vi "PISetAxisPos.vi"(0 "Position":sgl format="%.2f", 1 "Axis":i32) -> ()   [LabVIEW 2009]
uses:
  AO Update Channel (scaled value).vi
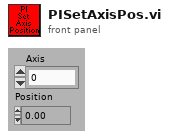
[diagram p1: front panel]
types:
  T1 = typedef "StageSettings.ctt" = cluster{"channels (x, y, z)":tag, "Stage Scaling (V/µm)":dbl}
  T2 = typedef "AnalogSettings.ctt" = cluster{"PCI 671x Device Number":u32, "Samples per Unit":u32}
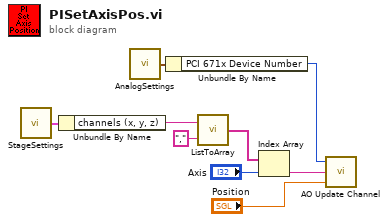
[diagram p0: block diagram]
diagram:
  n1 = call "StageSettings.vi"() -> ("PI Stage Setup (output)"=w9:T1)  [unwired: 2 in]
  n2 = Unbundle By Name(w9) -> ("channels (x, y, z)"=w6:tag)
  n3 = call "AnalogSettings.vi"() -> ("Analog Settings (output)"=w8:T2)  [unwired: 2 in]
  n4 = Unbundle By Name(w8) -> ("PCI 671x Device Number"=w7:u32)
  n5 = call "ListToArray.vi"("delimiter"=",", "list"=w6) -> ("Array"=w4:string[])
  n6 = Index Array(array=w4, index="Axis") -> (element=w2:string)
  n7 = call-poly "AO Update Channel.vi"("value"="Position", "channel (0)"=w2, "device"=w7) -> ()
